vi "Exp10 Identificação de Sistemas.vi"() -> ()   [LabVIEW 2017]
doc: "This example demonstrates a simple PID position controller for a Quanser SRV-02 plant."
uses:
  <vilib>/Simulation/Scripting/Companion Diagram/SimConfigNode/SimParams.ctl
  <vilib>/Simulation/Scripting/Companion Diagram/SimConfigNode/_simSolvers.ctl
  <vilib>/Simulation/Implementation/Shared/SIMSCR Execution Mode.ctl
  <vilib>/Platform/TimedLoop/XDataNode/timing_clust.ctl
  <vilib>/Platform/TimedLoop/XDataNode/nitl_modes.ctl
  <vilib>/Platform/TimedLoop/XDataNode/wakeup.ctl
  <vilib>/Simulation/Param Hierarchy/Typedefs/SIMPH Param Control Actions.ctl
  <vilib>/Simulation/Implementation/Shared/NILVSim_ParamChanged.vi
  <vilib>/Simulation/Implementation/Shared/NILVSim_FinishedLate.vi
  <vilib>/Simulation/Implementation/Shared/NILVSIM_BeginStep.vi
  <vilib>/Simulation/SignalArithmetic/Implementation/NILVSim Gain.llb/SIM Gain (scalar).vi
  <vilib>/Simulation/ContinuousLinear/Implementation/NILVSim Derivative.llb/SIM derivative (scalar).vi
  <vilib>/Simulation/Utility/Implementation/NILVSim Collector.llb/SIM Collector (scalar).vi
  <vilib>/Simulation/DataSources/Implementation/NILVSim Chirp Signal.llb/SIM Chirp Signal (scalar).vi
  <vilib>/Simulation/Nonlinear/Implementation/NILVSim Saturation.llb/SIM Saturation (scalar).vi
  <vilib>/Simulation/ContinuousLinear/Implementation/NILVSim Transfer Function.llb/SIM Transfer Function Distributor (SISO).vi
  <vilib>/Simulation/ContinuousLinear/Implementation/NILVSim Transfer Function.llb/SIM Transfer Function Collector (SISO).vi
  <vilib>/Simulation/Implementation/Shared/NILVSim_Manager.vi
  <vilib>/Utility/error.llb/Clear Errors.vi
  <vilib>/Simulation/Implementation/Shared/NILVSim_FinalizeModel.vi
  <vilib>/Simulation/Utility/Implementation/NILVSim Collector.llb/NILVSim Collector core (scalar).vi
  <vilib>/Simulation/Implementation/Shared/SIM Unbundle Sim Info.vi
  <vilib>/Simulation/Implementation/Shared/SIMSH Read Queue.vi
  <vilib>/Simulation/Implementation/Shared/NILVSim_Initialize.vi
  <vilib>/Simulation/Utility/Implementation/NILVSim Get Time and IsAcceptedStep.vi
  <vilib>/Simulation/Implementation/Shared/NILVSim_GetModelError.vi
  <vilib>/Simulation/Implementation/Shared/SIM Bundle Sim Info.vi
  <vilib>/addons/System Identification/Parametric Estimation.llb/SI Estimate Continuous Transfer Function Model (SISO Array).vi
  <vilib>/addons/Control Design/_Model Construction/Model Creation.llb/Model Creation SubVI/cd_Create Transfer Function Model.vi
  <vilib>/addons/Control Design/_Utility/Model Viewer.llb/Model Viewer SubVI/cd_Draw Transfer Function Equation (TF).vi
  <vilib>/Simulation/Scripting/Companion Diagram/SimConfigNode/SimDog.xnode
  <vilib>/Quanser/Rapid Control Prototyping Toolkit/hardware/HIL Immediate IO/_TypeSpecific/CL HIL Read Encoder (Scalar).vi
  <vilib>/Quanser/Rapid Control Prototyping Toolkit/hardware/HIL Immediate IO/CL HIL Read.vi
  <vilib>/Quanser/Rapid Control Prototyping Toolkit/hardware/HIL Immediate IO/_TypeSpecific/CL HIL Write Analog (Scalar).vi
  <vilib>/Quanser/Rapid Control Prototyping Toolkit/hardware/HIL Immediate IO/CL HIL Write.vi
  <vilib>/Platform/TimedLoop/XDataNode/XDataNode.xnode
  <vilib>/Simulation/Implementation/XNodeFramework/SimXNode/SimX.xnode
  <vilib>/Simulation/ContinuousLinear/Implementation/NILVSim Transfer Function.llb/SIM Transfer Function (SISO).vi
  <vilib>/addons/System Identification/NI_SysID.lvlib
  <vilib>/addons/Control Design/_Utility/NI_CD_Model Viewer.lvlib
  <vilib>/addons/Control Design/_Model Construction/NI_LinSys_Model Creation.lvlib
  <vilib>/Platform/TimedLoop/XDataNode/XDNodeRunTimeDep.lvlib
  <vilib>/Simulation/Implementation/Shared/NI_SIM_Implementation.lvlib
panel:
  in  "orders of transfer function model":cluster{" num order":i32, "den order":i32}={" num order"=1, "den order"=2}
  out "Equation":picture
  out "XY Graph":cluster{"Time":dbl[], "Signal":dbl[]}[](graph)=[{"Time"=[0.0, 0.01, 0.02, 0.03, 0.04, 0.05, 0.06, 0.07, 0.08, 0.09, 0.1, 0.11, 0.12, 0.13, 0.14, 0.15, 0.16, 0.17, 0.18, 0.19, 0.2, 0.21, 0.22, 0.23, 0.24, 0.25, 0.26, 0.27, 0.28, 0.29, 0.3, 0.31, 0.32, 0.33, 0.34, 0.35000000000000003, 0.36, 0.37, 0.38, 0.39, 0.4, 0.41000000000000003, 0.42, 0.43, 0.44, 0.45, 0.46, 0.47000000000000003, 0.48, 0.49, 0.5, 0.51, 0.52, 0.53, 0.54, 0.55, 0.56, 0.5700000000000001, 0.58, 0.59, 0.6, 0.61, 0.62, 0.63, 0.64, 0.65, 0.66, 0.67, 0.68, 0.6900000000000001, 0.7000000000000001, 0.71, 0.72, 0.73, 0.74, 0.75, 0.76, 0.77, 0.78, 0.79, 0.8, 0.81, 0.8200000000000001, 0.8300000000000001, 0.84, 0.85, 0.86, 0.87, 0.88, 0.89, 0.9, 0.91, 0.92, 0.93, 0.9400000000000001, 0.9500000000000001, 0.96, 0.97, 0.98, 0.99, 1.0, 1.01, 1.02, 1.03, 1.04, 1.05, 1.06, 1.07, 1.08, 1.09, 1.1, 1.11, 1.12, 1.1300000000000001, 1.1400000000000001, 1.1500000000000001, 1.16, 1.17, 1.18, 1.19, 1.2, 1.21, 1.22, 1.23, 1.24, 1.25, 1.26, 1.27, 1.28, 1.29, 1.3, 1.31, 1.32, 1.33, 1.34, 1.35, 1.36, 1.37, 1.3800000000000001, 1.3900000000000001, 1.4000000000000001, 1.41, 1.42, 1.43, 1.44, 1.45, 1.46, 1.47, 1.48, 1.49, 1.5, 1.51, 1.52, 1.53, 1.54, 1.55, 1.56, 1.57, 1.58, 1.59, 1.6, 1.61, 1.62, 1.6300000000000001, 1.6400000000000001, 1.6500000000000001, 1.6600000000000001, 1.67, 1.68, 1.69, 1.7, 1.71, 1.72, 1.73, 1.74, 1.75, 1.76, 1.77, 1.78, 1.79, 1.8, 1.81, 1.82, 1.83, 1.84, 1.85, 1.86, 1.87, 1.8800000000000001, 1.8900000000000001, 1.9000000000000001, 1.9100000000000001, 1.92, 1.93, 1.94, 1.95, 1.96, 1.97, 1.98, 1.99, 2.0, 2.0100000000000002, 2.02, 2.0300000000000002, 2.04, 2.05, 2.06, 2.07, 2.08, 2.09, 2.1, 2.11, 2.12, 2.13, 2.14, 2.15, 2.16, 2.17, 2.18, 2.19, 2.2, 2.21, 2.22, 2.23, 2.24, 2.25, 2.2600000000000002, 2.27, 2.2800000000000002, 2.29, 2.3000000000000003, 2.31, 2.32, 2.33, 2.34, 2.35, 2.36, 2.37, 2.38, 2.39, 2.4, 2.41, 2.42, 2.43, 2.44, 2.45, 2.46, 2.47, 2.48, 2.49, 2.5, 2.5100000000000002, 2.52, 2.5300000000000002, 2.54, 2.5500000000000003, 2.56, 2.57, 2.58, 2.59, 2.6, 2.61, 2.62, 2.63, 2.64, 2.65, 2.66, 2.67, 2.68, 2.69, 2.7, 2.71, 2.72, 2.73, 2.74, 2.75, 2.7600000000000002, 2.77, 2.7800000000000002, 2.79, 2.8000000000000003, 2.81, 2.82, 2.83, 2.84, 2.85, 2.86, 2.87, 2.88, 2.89, 2.9, 2.91, 2.92, 2.93, 2.94, 2.95, 2.96, 2.97, 2.98, 2.99, 3.0], "Signal"=[0.0, 0.0, 0.0, 0.0, 0.0, 0.0, 0.0, 0.0, 0.0, 0.0, 0.0, 0.0, 0.0, 0.0, 0.0, 0.0, 0.0, 0.0, 0.0, 0.0, 0.0, 0.0, 0.4601942363656932, 1.6106798272799223, 3.15233051910499, 5.243913323387068, 7.444332064569623, 9.720935961582514, 11.774752925857234, 14.040774426307783, 16.087183712988896, 17.97986445003133, 19.672896355053588, 21.31821292493486, 23.11420645476371, 24.46344077291706, 25.684021337443806, 26.906583121705143, 27.9464540652343, 29.134557962070396, 29.966230689855678, 30.732479293851647, 31.544969858468225, 32.20575210097304, 33.12849390709206, 33.31421893500966, 34.27257608001021, 33.654882219686684, 35.52346769928867, 35.8190502150056, 35.105569503276, 35.89467686688921, 36.81520741051106, 36.999384554680574, 37.864619333784425, 38.286205984610824, 38.673355487462395, 39.036398986731704, 39.29052943622016, 39.65249844540851, 39.905876751840225, 40.54343580270811, 40.621571749223094, 40.86034460632982, 41.02748560630459, 41.236523153560015, 41.75100482573141, 41.92706430170509, 42.050305934886666, 42.22861392538686, 42.445468366010196, 42.597266474446535, 42.70352515035206, 42.96198391803208, 43.050866208135, 43.20512265848014, 43.313102173721745, 43.388687834390865, 42.521209324127874, 42.92640168694835, 43.57819173001518, 43.758328218342555, 43.976462607444816, 44.4052732216359, 44.52136295702326, 44.51058692452156, 44.59508254904322, 45.29850141712047, 44.87050615204317, 44.84702600830835, 44.922628754967164, 44.88351183035525, 45.31632421949259, 44.882982113703655, 45.31595341783637, 45.25087794163679, 45.29736395557028, 43.94932145622669, 44.47831326305631, 44.75656868056394, 45.04338632009238, 45.15211982048909, 45.32027211803999, 45.8061341154182, 45.686043277217266, 45.69401853774971, 45.699601220122425, 45.70350909778332, 45.706244612145944, 45.70815947219979, 45.80153872151046, 45.86690419602815, 45.91266002819053, 45.94468911070398, 46.335264857556204, 46.24051249126017, 46.17418583485272, 46.12775717536804, 46.09525711372845, 46.072507070580535, 45.964543193104, 46.34916271523622, 46.250240991636176, 46.273034632389134, 46.56510672273581, 45.11285793506171, 45.38482764551403, 45.66724529010363, 45.864937641316565, 46.00332228716541, 46.00815269198661, 46.10357282263444, 46.44648345590752, 46.41040435737908, 46.293110141136175, 46.30304303703914, 46.21795721689822, 46.61859137916516, 46.53087990365964, 46.46948187080556, 46.51854209508091, 46.46084540480045, 46.78861311069725, 46.64989511573189, 46.55279251925614, 46.48482070172332, 46.34520158217715, 46.33950704576782, 46.335520870281286, 46.33273054744093, 46.33077732145246, 45.31698274325617, 45.61975385852313, 45.831693639210215, 46.07209033296417, 46.14832917131873, 46.56985174725952, 46.496762161325684, 46.81375484026439, 46.299338937336294, 46.675558583472025, 46.57075694667423, 46.49739580091577, 46.44604299888507, 46.41009603746336, 46.47697201174137, 46.43174634646298, 46.4921272280411, 46.81051038696549, 46.66522320911966, 46.655561031900774, 46.556758660574566, 46.487597000646005, 46.43918383869624, 46.40529462533118, 46.381572175975634, 46.364966461426974, 46.3533424612429, 45.33277834110927, 45.72284962429329, 45.99589952252253, 46.46315099310239, 46.422071633415484, 46.48535492890764, 46.80576977757197, 46.66190478254419, 46.561199286024745, 46.85886082755394, 46.69906851753157, 46.58721390051592, 46.50891566860538, 46.454106906267576, 45.49535229989953, 45.744612548174224, 46.01113356923876, 46.19769828398436, 46.23625473703286, 46.263244254166814, 46.374175763433996, 46.72794436173999, 46.60742699146181, 46.5230648322675, 46.46401132083075, 46.42267386282565, 46.39373764222146, 46.37348228779914, 46.819497776069326, 46.763553228765446, 46.63235319837993, 46.63255202438287, 46.540652355312126, 46.84447797605479, 46.781039368755465, 46.64459349637233, 46.54908138570476, 46.48222290823726, 45.05483926491321, 45.80440881277512, 45.960952107186706, 46.07053241327462, 46.23927747480935, 46.35739901788346, 46.716200639854925, 46.691245233415366, 46.581737601634885, 46.50508225938792, 46.543462367089084, 46.478289595205865, 46.80082404398104, 46.65844276903023, 46.558775876565285, 46.489009051839204, 46.808327663624375, 46.755734150054174, 46.626879843281856, 46.62872067581441, 46.630009258586995, 46.53887241925502, 46.47507663172202, 46.52245842772295, 46.46358683764957, 46.42237672459883, 46.39352964546268, 46.373336690068, 46.35920162129153, 45.3368797531436, 45.725720612717005, 45.90587036714645, 46.124014042519, 46.276714615280845, 46.65972155803246, 46.559671028866845, 46.581674505723704, 46.505038092250714, 46.819547991911804, 46.67154953258238, 46.56795061105117, 46.86358675507276, 46.702376666795054, 46.58952960500004, 46.60257550901756, 45.23112493273186, 45.92780878024924, 46.139370931690955, 46.195425590427796, 46.23466385154339, 46.63028602341688, 46.63110500190873, 46.815755981399626, 46.66889512522324, 46.65813137317381, 46.55855789946517, 46.48885646786974, 46.80822085484512, 46.75565938390869, 46.718866354253, 46.60107238622122, 46.610655455871765, 46.52532475735436, 46.92578750475734, 44.99717909338446, 45.76404669270543, 45.93269862313792, 46.050754974440665, 46.13339442035197, 46.191242032490926, 46.32377420826013, 46.32450788402622, 46.78521569342764, 46.64751692364389, 46.643166632067214, 46.916237969783985, 46.831271364365286, 46.67975589329982, 46.57369506355381, 46.49945248273178, 46.44748267615575, 46.77925920064597, 46.64334737869567, 46.64024795060408, 46.54603950366679]}, ...(2 in all)]
  out "Degrau (V)":dbl(graph)=2.0
  out "Velocidade (rad/s)":dbl(graph)=46.54603950366679
  out "encoder counts":i32=39739
  out "Error":errorcluster
  # "IDENTIFICA敲O MOTOR DC"
  # "Caracterização do Motor DC \nutilizando o kit Qube Servo- 2 \nda Quanser"
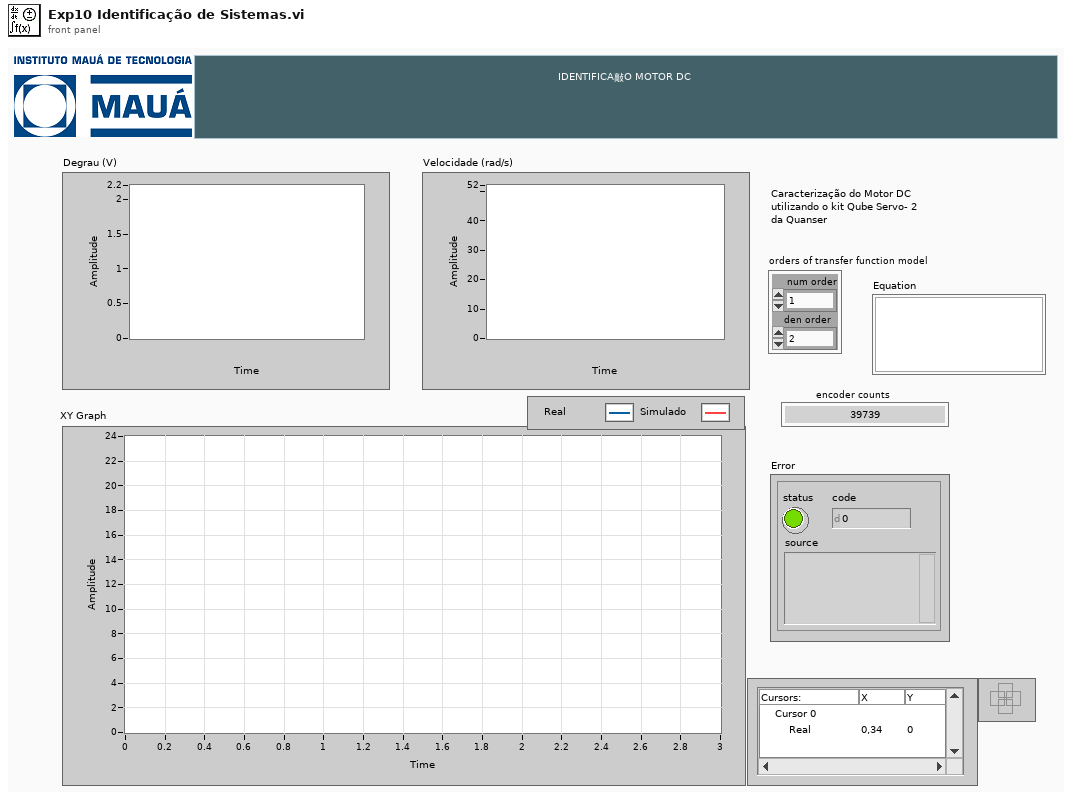
[diagram p1: front panel]
types:
  T1 = typedef "NI_LinSys_Model Typedefs.lvlib/CD Transfer Function Model (MIMO).ctl" = cluster{"properties":T2, "transfer function(s)":T3[][]}
  T2 = typedef "NI_LinSys_Model Typedefs.lvlib/CD General Elements.ctl" = cluster{"Model name":string, "Input names":string[], "Output names":string[], "Input Delays":dbl[], "Output Delays":dbl[], "Sampling Time":dbl, "Notes":string}
  T3 = typedef "NI_LinSys_Model Typedefs.lvlib/CD Transfer Function Model (SISO).ctl" = cluster{"Numerator":dbl[], "Denominator":dbl[], "delay":dbl}
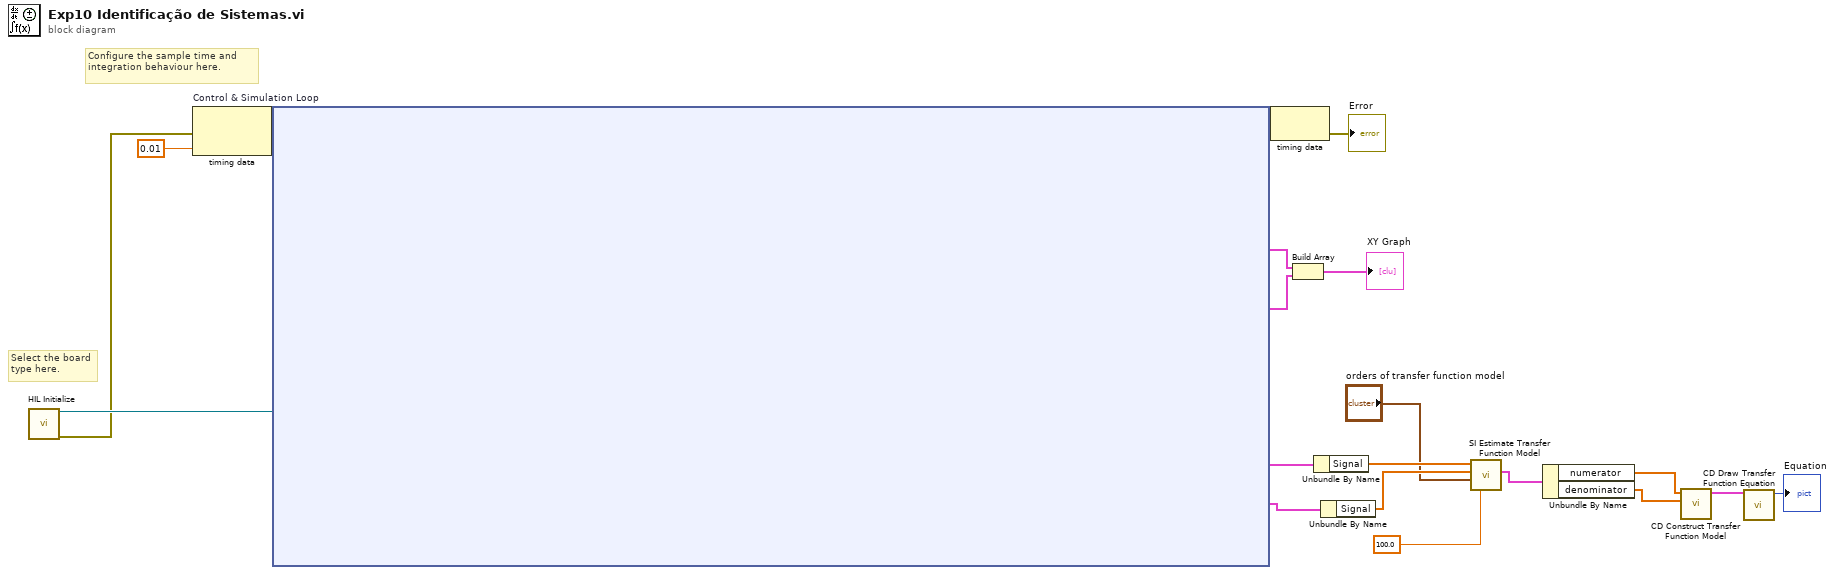
[diagram p0: block diagram]
diagram:
  # "Configure the sample time and integration behaviour here."
  # "Select the board\ntype here."
  n1 = call "HIL Initialize"() -> ("board out"=w18:refnum<class "HIL Board.lvclass">, "error out"=w15:errorcluster)  [unwired: 14 in]
  n2 = node-c288(w15, 0.01 ("Step Size (s)")) -> (w20:variant)
  n3 = node-c254 "Control & Simulation Loop"(w20, w18) -> (w19:variant, w14:cluster{"Time":dbl[], "Signal":dbl[]}, w13:cluster{"Time":dbl[], "Signal":dbl[]}, w5:cluster{"Time":dbl[], "Signal":dbl[]}, w11:cluster{"Time":dbl[], "Signal":dbl[]})
  n4 = node-c288(w19) -> (→"Error":errorcluster)
  n5 = Build Array "Build Array"(w14, w13) -> (→"XY Graph":cluster{"Time":dbl[], "Signal":dbl[]}[])
  n6 = Unbundle By Name(w5) -> ("Signal"=w3:dbl[])
  n7 = Unbundle By Name(w11) -> ("Signal"=w2:dbl[])
  n8 = call-poly <vilib>:"SI Estimate Transfer Function Model.vi"("sampling rate (Hz)"=100.0, "orders of transfer function model"="orders of transfer function model", "response signal"=w2, "stimulus signal"=w3) -> ("coefficients of transfer function model"=w10:cluster{"numerator":dbl[], "denominator":dbl[]})  [unwired: 4 in, 3 out]
  n9 = Unbundle By Name(w10) -> ("numerator"=w9:dbl[], "denominator"=w8:dbl[])
  n10 = call-poly <vilib>:"CD Construct Transfer Function Model.vi"("Denominator"=w8, "Numerator"=w9) -> ("Transfer Function Model"=w7:T1)  [unwired: 8 in, 1 out]
  n11 = call-poly <vilib>:"CD Draw Transfer Function Equation.vi"("Transfer Function Model"=w7) -> ("Equation"=→"Equation":picture)  [unwired: 8 in, 2 out]
